vi "Day 3 Puzzle 1.vi"() -> ()   [LabVIEW 2021]
uses:
  <vilib>/Utility/file.llb/Read Delimited Spreadsheet (string).vi
panel:
  out "Sum":i32
  in  "File Path":path
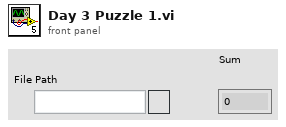
[diagram p1: front panel]
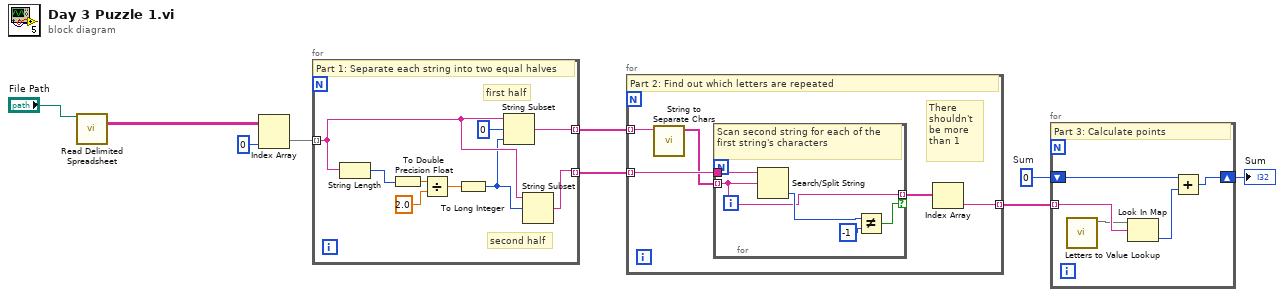
[diagram p0: block diagram]
diagram:
  w2 = 0  # Sum
  n1 = call-poly <vilib>:"Read Delimited Spreadsheet.vi"("file path (dialog if empty)"="File Path") -> ("all rows"=w8:string[][])  [unwired: 9 in, 5 out]
  n2 = Index Array(array=w8, index (col)=0 ("disabled index (col)")) -> (element=w6:string[])  [unwired: 1 in]
  n3 = for {
    tunnel: w6 -> [w14] mode=indexing
    tunnel: [w11] -> w4 mode=indexing
    tunnel: [w10] -> w5 mode=indexing
    # "second half"
    # "first half"
    # "Part 1: Separate each string into two equal halves"
    n4 = String Length(string=w14) -> (length=w12:i32)
    n5 = To Double Precision Float(number=w12) -> (double precision float=w17:dbl)
    n6 = Divide(x=w17, y=2.0) -> (x/y=w16:dbl)
    n7 = To Long Integer(number=w16) -> (32bit integer=w13:i32)
    n8 = String Subset(string=w14, offset (0)=0, length (rest)=w13) -> (substring=w11:string)
    n9 = String Subset(string=w14, offset (0)=w13) -> (substring=w10:string)  [unwired: 1 in]
  }
  n10 = for {
    tunnel: w4 -> [w23] mode=indexing
    tunnel: w5 -> [w22] mode=indexing
    tunnel: [w20] -> w3 mode=indexing
    # "There\nshouldn't \nbe more\nthan 1"
    # "Part 2: Find out which letters are repeated"
    n11 = call "String to Separate Chars.vi"("String"=w23) -> ("Array"=w21:string[])  [unwired: 10 in]
    n12 = for {
      tunnel: w22 -> [w25]
      tunnel: w21 -> [w24] mode=indexing
      tunnel: [w24] -> w19 mode=indexing if=w27
      # "Scan second string for each of the first string's characters"
      n13 = Search/Split String(string=w25, search string/char (-)=w24) -> (offset of match=w26:i32)  [unwired: 1 in, 2 out]
      n14 = Not Equal?(x=w26, y=-1) -> (x != y?=w27:bool)
    }
    n15 = Index Array(array=w19) -> (element=w20:string)  [unwired: 1 in]
  }
  n16 = for {
    tunnel: w3 -> [w33] mode=indexing
    shift-right: [w29] -> w1
    shift-left: w2 -> [w31]
    # "Part 3: Calculate points"
    n17 = call "Letters to Value Lookup.vi"() -> ("map in"=w32:map{string, i32})  [unwired: 11 in]
    n18 = Look In Map(map=w32, key=w33) -> (value=w30:i32)  [unwired: 1 in, 1 out]
    n19 = Add(x=w31, y=w30) -> (x+y=w29:i32)
  }
  "Sum" <- w1
